vi "Zadanie5.vi"() -> ()   [LabVIEW 2011]
panel:
  out "Waveform Chart":dbl(graph)
  out "Tank":dbl(slide) scale=0.0..20.0
  in  "stop":bool
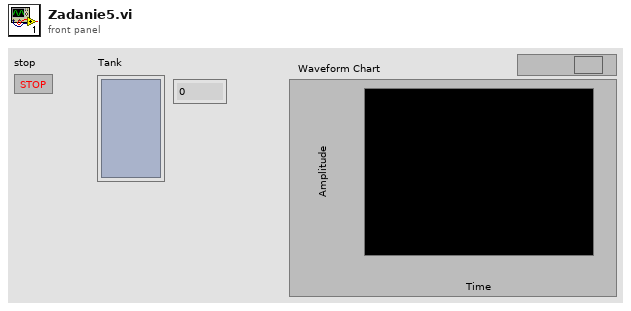
[diagram p1: front panel]
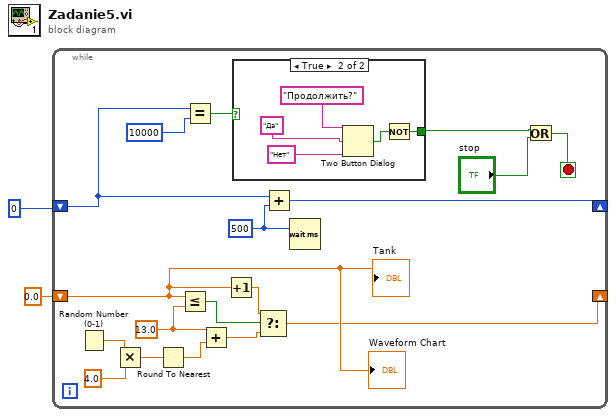
[diagram p0: block diagram]
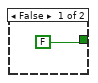
[diagram p2: hidden frame]
diagram:
  n1 = while {
    shift-right: [w12] -> _
    shift-left: 0.0 -> [w13]
    shift-right: [w6] -> _
    shift-left: 0 -> [w7]
    stop <- w5 stop-if-true
    w8 = 500
    w16 = 13.0
    n2 = Random Number (0-1)() -> (number: 0 to 1=w14:dbl)
    n3 = Multiply(x=w14, y=4.0) -> (x*y=w20:dbl)
    n4 = Round To Nearest(number=w20) -> (nearest integer value=w19:dbl)
    n5 = Less Or Equal?(x=w13, y=w16) -> (x <= y?=w11:bool)
    n6 = Equal?(x=w7, y=10000) -> (x = y?=w9:bool)
    n7 = Add(x=w16, y=w19) -> (x+y=w18:dbl)
    n8 = Increment(x=w13) -> (x+1=w17:dbl)
    n9 = case shown="True" w9 {
      tunnel: [FALSE w22] -> w3
      frame False {
      }
      frame True {
        n10 = Two Button Dialog(message="Продолжить?", 1:"Нет", 2:"Да") -> (T button?=w23:bool)
        n11 = Not(x=w23) -> (.not. x?=w22:bool)
      }
    }
    n12 = Select(t=w17, s=w11, f=w18) -> (s? t:f=w12:dbl)
    n13 = Add(x=w7, y=w8) -> (x+y=w6:i32)
    n14 = Wait (ms)(milliseconds to wait=w8) -> ()  [unwired: 1 out]
    n15 = Or(x=w3, y="stop") -> (x .or. y?=w5:bool)
    "Tank" <- w13
    "Waveform Chart" <- w13
  }
